vi "NI2564BDisconnectAll.vi"(8 "error in (no error)":errorcluster, 10 "gRPCid":T4, 11 "HVC9 In":T1) -> (0 "error out":errorcluster, 3 "HVC9 Out":T1)   [LabVIEW 2019, in "HVC9 User.lvlib"]
uses:
  HVC9 User.lvlib
  Servers/HVC9/gRPC lvSupport/Server API/typeDefs/grpcId.ctl
  Types/HVC9.ctl
  Types/HVC9 gRPC IDs.ctl
  Types/HVC9 Data.ctl
  Servers/HVC9/HVC9 Class/RPC Messages/measurementservice_NI2564DisconnectAllResponse/measurementservice_NI2564DisconnectAllResponse_Data.ctl
  Servers/HVC9/HVC9 Class/RPC Messages/measurementservice_ErrorOut/measurementservice_ErrorOut_Data.ctl
  Servers/HVC9/HVC9 Class/HVC9.lvclass
  Servers/HVC9/gRPC lvSupport/gprc-lvsupport.lvlib
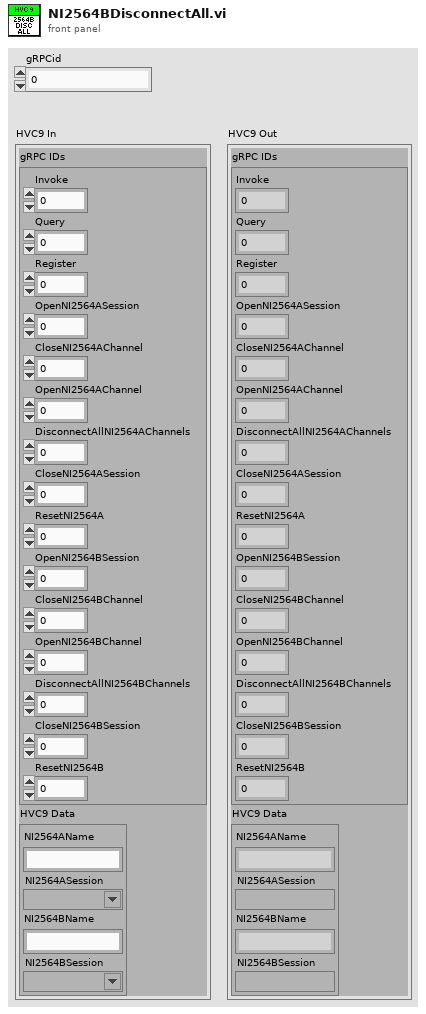
[diagram p1: front panel]
types:
  T1 = typedef "HVC9 User.lvlib/HVC9.ctl" = cluster{"gRPC IDs":T2, "HVC9 Data":T3}
  T2 = typedef "HVC9 User.lvlib/HVC9 gRPC IDs.ctl" = cluster{"Invoke ":u32, "Query":u32, "Register":u32, "OpenNI2564ASession":u32, "CloseNI2564AChannel ":u32, "OpenNI2564AChannel":u32, "DisconnectAllNI2564AChannels":u32, "CloseNI2564ASession":u32, "ResetNI2564A":u32, "OpenNI2564BSession":u32, "CloseNI2564BChannel ":u32, "OpenNI2564BChannel":u32, "DisconnectAllNI2564BChannels":u32, "CloseNI2564BSession":u32, "ResetNI2564B":u32}
  T3 = typedef "HVC9 User.lvlib/HVC9 Data.ctl" = cluster{"NI2564AName":string, "NI2564ASession":refnum<k15>, "NI2564BName":string, "NI2564BSession":refnum<k15>}
  T4 = typedef "HVC9.lvlib/gprc-lvsupport.lvlib/grpcId.ctl" = u64
  T5 = typedef "HVC9.lvlib/HVC9.lvclass/measurementservice_ErrorOut_Data.ctl" = cluster{"errCode":i32, "errMessage":string}
  T6 = typedef "HVC9.lvlib/HVC9.lvclass/measurementservice_NI2564DisconnectAllResponse_Data.ctl" = cluster{"error":T5}
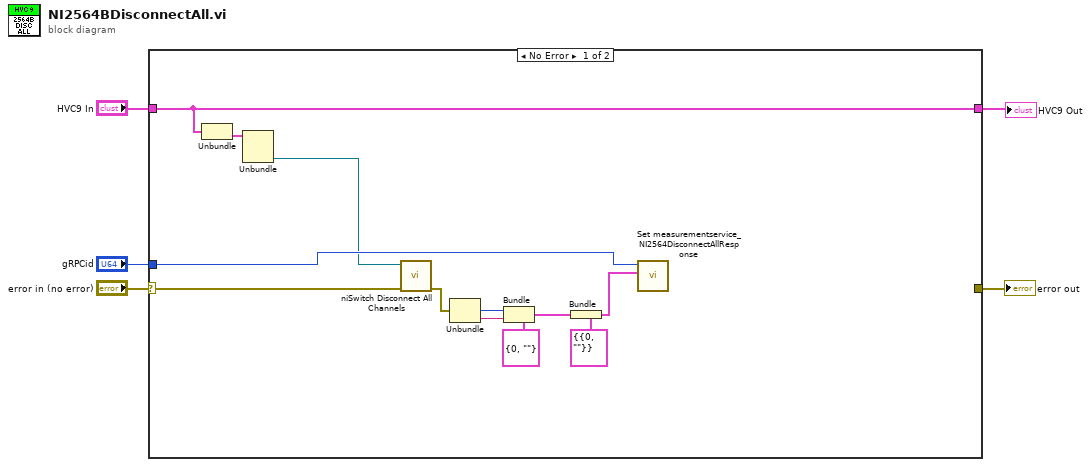
[diagram p0: block diagram]
diagram:
  n1 = case shown="No Error" "error in (no error)" {
    selector: "error in (no error)" -> [w14 w18]
    tunnel: [w13 w19] -> w1
    tunnel: "HVC9 In" -> [w13 w19]
    tunnel: "gRPCid" -> [w12 _]
    tunnel: [_ w18] -> w4
    frame No Error {
      n2 = Unbundle(w13) -> ("HVC9 Data"=w15:T3)  [unwired: 1 out]
      n3 = Unbundle(w15) -> ("NI2564BSession"=w6:refnum<k15>)  [unwired: 3 out]
      n4 = call <instrlib>:"niSwitch Disconnect All Channels.vi"("error in (no error)"=w14, "instrument handle"=w6) -> ("error out"=w10:errorcluster)  [unwired: 8 in, 1 out]
      n5 = Unbundle(w10) -> ("code"=w16:i32, "source"=w17:string)  [unwired: 1 out]
      n6 = Bundle(cluster=T5 {"errCode"=0, "errMessage"=""} ("error"), "errCode"=w16, "errMessage"=w17) -> (w7:T5)
      n7 = Bundle(cluster=T6 {"error"={"errCode"=0, "errMessage"=""}} ("measurementservice_NI2564DisconnectAllResponse_Data"), "error"=w7) -> (w11:T6)
      n8 = call "Set measurementservice_NI2564DisconnectAllResponse.vi"("Message Data"=w11, "gRPCid"=w12) -> ()  [unwired: 9 in, 1 out]
    }
    frame Error {
    }
  }
  "error out" <- w4
  "HVC9 Out" <- w1
